vi "timing.vi"() -> ()   [LabVIEW 2018]
panel:
  in  "phase 4":u32
  in  "phase 3":u32
  in  "phase 2":i8
  in  "phase 1":u32
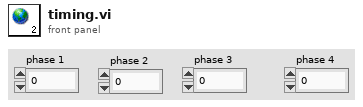
[diagram p1: front panel]
diagram:
